vi "tcp-ip RPI3.vi"() -> ()   [LabVIEW 2015]
panel:
  out "?":dbl
  out "Thermometer":dbl(slide) scale=0.0..100.0
  out "Waveform Chart":dbl(graph)
  in  "?":bool
  out "LECTURA RASPBERRY":string
  in  "PUERTO":u16
  in  "DIRECCION IP:":string
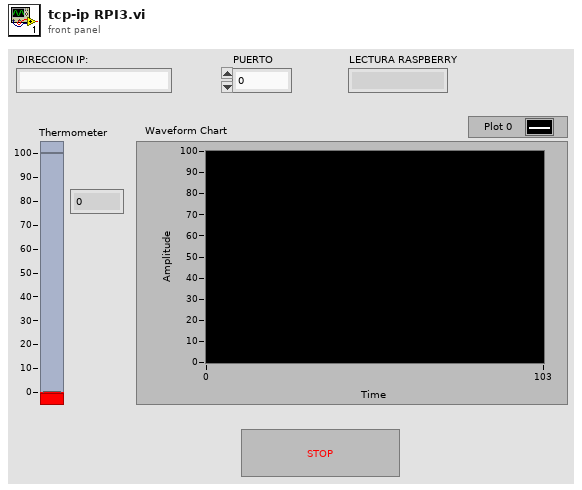
[diagram p1: front panel]
types:
  T1 = enum16{"Standard", "Buffered", "CRLF", "Immediate"}
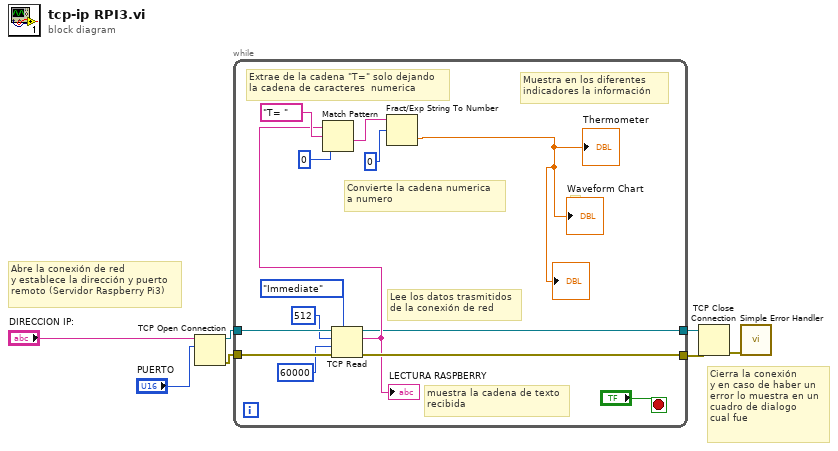
[diagram p0: block diagram]
diagram:
  # "Cierra la conexión\ny en caso de haber un \nerror lo muestra en un\ncuadro de dialogo \ncual fue"
  # "Abre la conexión de red \ny establece la dirección y puerto\nremoto (Servidor Raspberry Pi3)"
  n1 = TCP Open Connection(address="DIRECCION IP:", remote port or service name="PUERTO") -> (connection ID=w7:refnum<k5>, error out=w6:errorcluster)  [unwired: 3 in]
  n2 = while {
    tunnel: w7 -> [w21]
    tunnel: w6 -> [w20]
    tunnel: [w14] -> w5
    tunnel: [w9] -> w1
    stop <- "?" stop-if-true
    # "3"
    # "Muestra en los diferentes\nindicadores la información"
    # "Convierte la cadena numerica\na numero"
    # "Extrae de la cadena \"T=\" solo dejando\nla cadena de caracteres  numerica"
    # "muestra la cadena de texto\nrecibida"
    # "Lee los datos trasmitidos\nde la conexión de red"
    n3 = TCP Read(connection ID=w21, bytes to read=512, error in (no error)=w20, 7:T1."Immediate" ("mode (standard)"), 9:60000 ("timeout ms (25000)")) -> (connection ID out=w9:refnum<k5>, data out=w13:string, error out=w14:errorcluster)
    "LECTURA RASPBERRY" <- w13
    n4 = Match Pattern(string=w13, regular expression="T= ", offset (0)=0) -> (after substring=w11:string)  [unwired: 3 out]
    n5 = Fract/Exp String To Number(string=w11, offset=0) -> (number=→"Waveform Chart" →"Thermometer" →"?":dbl)  [unwired: 2 in, 1 out]
  }
  n6 = TCP Close Connection(connection ID=w1, error in (no error)=w5) -> (error out=w4:errorcluster)  [unwired: 1 in, 1 out]
  n7 = call <vilib>:"Simple Error Handler.vi"("error in (no error)"=w4) -> ()  [unwired: 4 in, 5 out]
